vi "Construct Path Component.vi"(11 "Segments":string[](array[string])) -> (2 "valid":bool, 3 "path":string)   [LabVIEW 2013, in "openURI.lvlib"]
uses:
  openURI.lvlib
  components/path/URI-Component.Path.lvclass
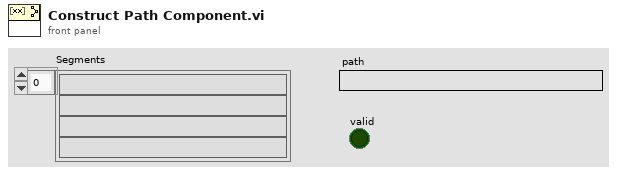
[diagram p1: front panel]
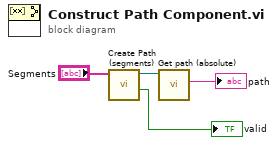
[diagram p0: block diagram]
diagram:
  n1 = call "Create Path (segments).vi"("Segments"="Segments") -> ("Valid"=→"valid":bool, "URI-Component.Path"=w3:refnum<class "URI-Component.Path.lvclass">)  [unwired: 7 in, 2 out]
  n2 = call "Get path (absolute).vi"("URI-Component.Path in"=w3) -> ("path-component"=→"path":string)  [unwired: 8 in, 2 out]
